vi "Calculate Vertices Array.vi"(8 "error in (no error)":errorcluster, 10 "2D Plotmatrix Datatype.lvclass in":refnum<class "XY Plot Matrix Datatype.lvclass">, 11 "Matrix Representation Array":T2[][](array[typedef])) -> (0 "error out":errorcluster, 1 "Max Range Array":T1[][](array[typedef]), 2 "2D Plotmatrix Datatype.lvclass out":refnum<class "XY Plot Matrix Datatype.lvclass">, 3 "Matrix Representation Array":T2[][](array[typedef]))   [LabVIEW 2017, in "XY Plot Matrix Datatype.lvclass"]
uses:
  <vilib>/Math Plots/2D Math Plots/XY Plot Matrix/XY Plot Matrix Datatype/XY Plot Matrix Datatype.lvclass
  <vilib>/Math Plots/2D Math Plots/XY Plot Matrix/XY Plot Matrix/Typedef/Matrix Representation.ctl
  <vilib>/Math Plots/2D Math Plots/2D Plot/2D Plot/Typedef/Range Cluster.ctl
  <vilib>/Math Plots/2D Math Plots/XY Plot Matrix/XY Plot Matrix Datatype/XY Plot Matrix Datatype.lvclass/XY Plot Matrix Datatype.ctl
  <vilib>/Math Plots/2D Math Plots/2D Plot/2D Plot/2D Plot.lvclass
  <vilib>/Math Plots/2D Math Plots/XY Plot Matrix/XY Plot Matrix/XY Plot Matrix.lvclass
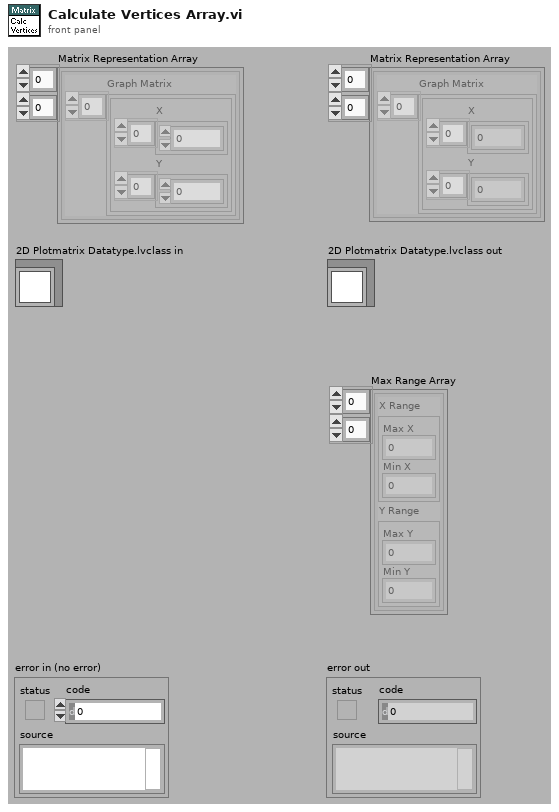
[diagram p1: front panel]
types:
  T1 = typedef "2D Plot.lvclass/Range Cluster.ctl" = cluster{"X Range":cluster{"Max X":dbl, "Min X":dbl}, "Y Range":cluster{"Max Y":dbl, "Min Y":dbl}}
  T2 = typedef "XY Plot Matrix.lvclass/Matrix Representation.ctl" = cluster{"Graph Matrix":cluster{"X":dbl[], "Y":dbl[]}[]}
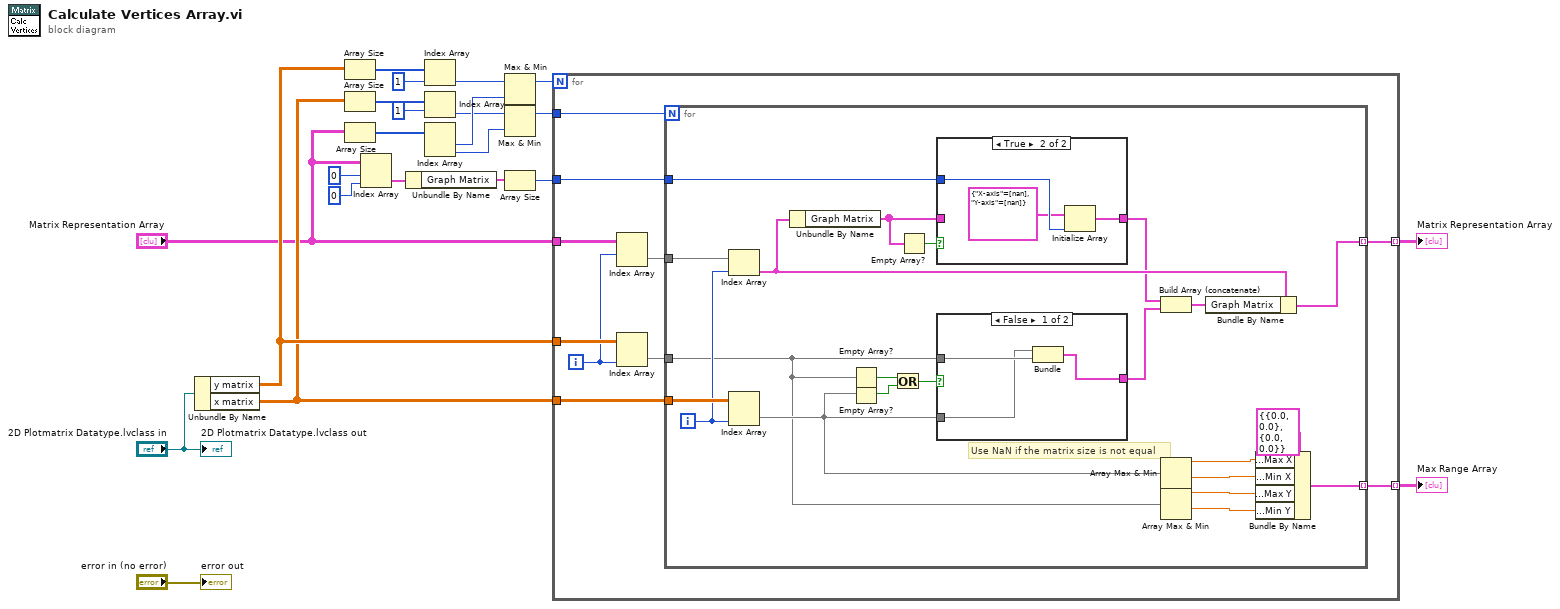
[diagram p0: block diagram]
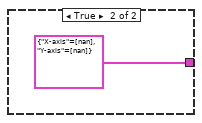
[diagram p3: hidden frame]
diagram:
  n1 = Unbundle By Name("2D Plotmatrix Datatype.lvclass in") -> ("y matrix"=w17:dbl[][], "x matrix"=w16:dbl[][])
  n2 = Array Size(array=w17) -> (size(s)=w21:i32[])
  n3 = Array Size(array=w16) -> (size(s)=w20:i32[])
  n4 = Array Size(array="Matrix Representation Array") -> (size(s)=w14:i32[])
  n5 = Index Array(array="Matrix Representation Array", index (row)=0, index (col)=0 ("disabled index (col)")) -> (element=w4:T2)
  n6 = Unbundle By Name(w4) -> ("Graph Matrix"=w3:cluster{"X":dbl[], "Y":dbl[]}[])
  n7 = Index Array(array=w21, index=1) -> (element=w12:i32)
  n8 = Index Array(array=w20, index=1) -> (element=w10:i32)
  n9 = Index Array(array=w14) -> (element #1=w13:i32, element #2=w9:i32)  [unwired: 2 in]
  n10 = Max & Min(x=w12, y=w13) -> (max(x,y)=w11:i32)  [unwired: 1 out]
  n11 = Max & Min(x=w10, y=w9) -> (max(x,y)=w8:i32)  [unwired: 1 out]
  n12 = Array Size(array=w3) -> (size(s)=w2:i32)
  n13 = for {
    N: w11 -> [_]
    tunnel: w17 -> [w32]
    tunnel: w16 -> [w31]
    tunnel: w8 -> [w33]
    tunnel: "Matrix Representation Array" -> [w28]
    tunnel: [w29] -> w15 mode=indexing
    tunnel: w2 -> [w25]
    tunnel: [w24] -> w1 mode=indexing
    i -> [w27]
    n14 = Index Array(array=w28, index (row)=w27) -> (element=w26:T2[])  [unwired: 1 in]
    n15 = Index Array(array=w32, index (col)=w27) -> (element=w30:dbl[])  [unwired: 1 in]
    n16 = for {
      N: w33 -> [_]
      tunnel: w31 -> [w55]
      tunnel: w30 -> [w40]
      tunnel: [w52] -> w29 mode=indexing
      tunnel: w26 -> [w51]
      tunnel: w25 -> [w45]
      tunnel: [w39] -> w24 mode=indexing
      i -> [w50]
      # "Use NaN if the matrix size is not equal"
      n17 = Index Array(array=w51, index=w50) -> (element=w49:T2)
      n18 = Index Array(array=w55, index (col)=w50) -> (element=w41:dbl[])  [unwired: 1 in]
      n19 = Unbundle By Name(w49) -> ("Graph Matrix"=w42:cluster{"X":dbl[], "Y":dbl[]}[])
      n20 = Empty Array?(array=w40) -> (empty?=w47:bool)
      n21 = Empty Array?(array=w41) -> (empty?=w48:bool)
      n22 = Or(x=w47, y=w48) -> (x .or. y?=w46:bool)
      n23 = Empty Array?(array=w42) -> (empty?=w44:bool)
      n24 = case shown="True" w44 {
        tunnel: w45 -> [_ w59]
        tunnel: [w56 w57] -> w43
        tunnel: w42 -> [w56 _]
        frame False {
        }
        frame True {
          n25 = Initialize Array(cluster{"X-axis":dbl[], "Y-axis":dbl[]} {"X-axis"=[nan], "Y-axis"=[nan]}, w59) -> (w57:cluster{"X-axis":dbl[], "Y-axis":dbl[]}[])
        }
      }
      n26 = case shown="False" w46 {
        tunnel: [w62 cluster{"X-axis":dbl[], "Y-axis":dbl[]} {"X-axis"=[nan], "Y-axis"=[nan]}] -> w54
        tunnel: w40 -> [w61 _]
        tunnel: w41 -> [w60 _]
        frame False {
          n27 = Bundle("x matrix"=w60, "y matrix"=w61) -> (w62:cluster{"x matrix":dbl[], "y matrix":dbl[]})  [unwired: 1 out]
        }
        frame True {
        }
      }
      n28 = Build Array (concatenate)(w43, w54) -> (w53:cluster{"X-axis":dbl[], "Y-axis":dbl[]}[])
      n29 = Array Max & Min(array=w41) -> (max value=w37:dbl, min value=w36:dbl)  [unwired: 2 out]
      n30 = Array Max & Min(array=w40) -> (max value=w35:dbl, min value=w34:dbl)  [unwired: 2 out]
      n31 = Bundle By Name(cluster=w49, "Graph Matrix"=w53) -> (w52:T2)
      n32 = Bundle By Name(cluster=T1 {"X Range"={"Max X"=0.0, "Min X"=0.0}, "Y Range"={"Max Y"=0.0, "Min Y"=0.0}} ("Max Range"), "X Range.Max X"=w37, "X Range.Min X"=w36, "Y Range.Max Y"=w35, "Y Range.Min Y"=w34) -> (w39:T1)
    }
  }
  "Matrix Representation Array" <- w15
  "Max Range Array" <- w1
  "2D Plotmatrix Datatype.lvclass out" <- "2D Plotmatrix Datatype.lvclass in"
  "error out" <- "error in (no error)"
